vi "Kinect Controls Overwrite(SubVI).vi"(8 "error in (no error)":errorcluster, 10 "Control cluster In":T1, 11 "Land/Take off In":bool) -> (0 "error out":errorcluster, 1 "Control cluster Out":T1, 2 "Hover Out":bool, 3 "Land/take off Out":bool)   [LabVIEW 2014]
uses:
  Kinect Global.vi
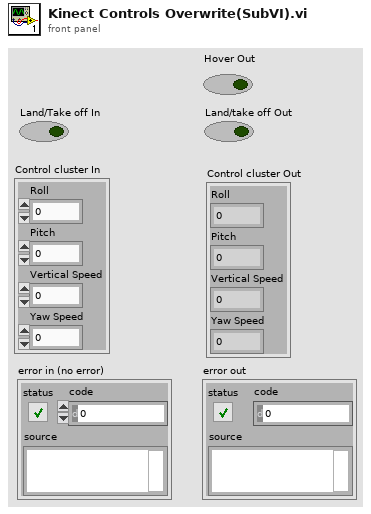
[diagram p1: front panel]
types:
  T1 = cluster{"Roll":dbl, "Pitch":dbl, "Vertical Speed":dbl, "Yaw Speed":dbl}
  T2 = typedef "Control cluster.ctl" = cluster{"Roll":sgl, "Pitch":sgl, "Vertical Speed":sgl, "Yaw Speed":sgl}
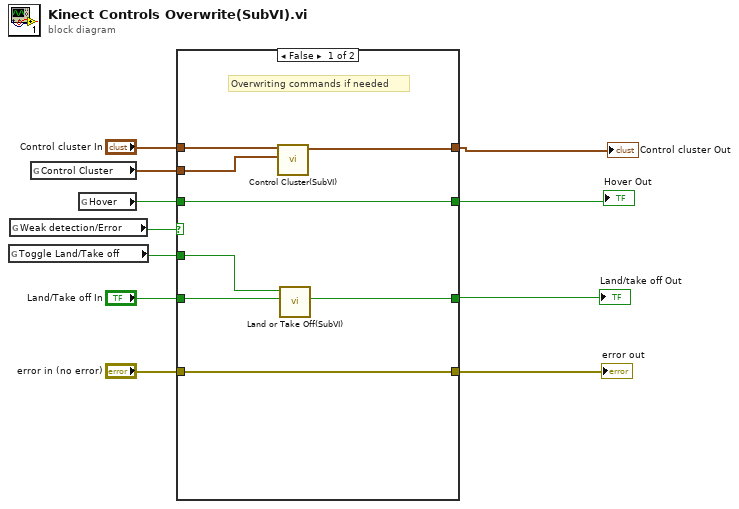
[diagram p0: block diagram]
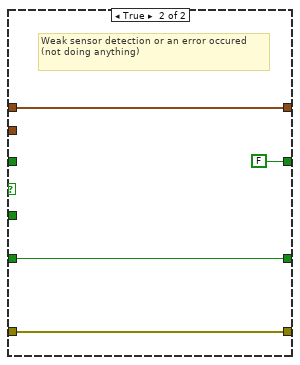
[diagram p2: hidden frame]
diagram:
  n1 = global read "Kinect Global.vi" "Toggle Land/Take off"() -> (w9:bool)
  n2 = global read "Kinect Global.vi" "Weak detection/Error"() -> (w8:bool)
  n3 = global read "Kinect Global.vi" "Control Cluster"() -> (w5:T2)
  n4 = global read "Kinect Global.vi" "Hover"() -> (w6:bool)
  n5 = case shown="False" w8 {
    tunnel: [w19 w21] -> w11
    tunnel: "Land/Take off In" -> [w18 w21]
    tunnel: w9 -> [w17 _]
    tunnel: "Control cluster In" -> [w15 w23]
    tunnel: [w13 w23] -> w2
    tunnel: w6 -> [w16 _]
    tunnel: [w16 FALSE ("Hover")] -> w1
    tunnel: w5 -> [w14 _]
    tunnel: "error in (no error)" -> [w12 w20]
    tunnel: [w12 w20] -> w3
    frame False {
      # "Overwriting commands if needed"
      n6 = call "Control Cluster(SubVI).vi"("Control cluster In New"=w14, "Control cluster In Original"=w15) -> ("Control cluster Out"=w13:T1)  [unwired: 9 in]
      n7 = call "Land or Take Off(SubVI).vi"("Land/Take off In"=w18, "Toggle Land/Take off"=w17) -> ("Boolean"=w19:bool)  [unwired: 9 in]
    }
    frame True {
      # "Weak sensor detection or an error occured (not doing anything)"
    }
  }
  "error out" <- w3
  "Land/take off Out" <- w11
  "Hover Out" <- w1
  "Control cluster Out" <- w2
